vi "ADAM_Server_Channels.vi"() -> (0 "DAQ Error":errorcluster)   [LabVIEW 2015]
uses:
  ADAM Client/Sub VIs/ADAM Controls/Search_mode.ctl
  <vilib>/Analysis/baseanly.llb/Mean (DBL).vi
  Globals/Meas_global.vi
  Globals/Trav_pos_global.vi
  <vilib>/Analysis/NI_AALBase.lvlib
panel:
  out "Waveform Graph":dbl[][](graph)
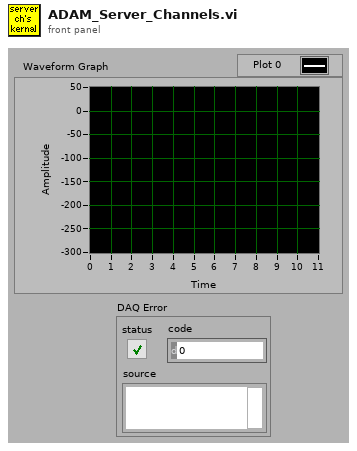
[diagram p1: front panel]
types:
  T1 = typedef "Analysis_info_cluster.ctl" = cluster{"Colour":u32, "Inst type":T2, "Inst name":string, "Symbol":string, "Code name":string, "Extra Info":string, "Inst Array":T3, "Extra Titles":string[], "Extra Values":string[], "U":dbl, "u^2":dbl, "u^3":dbl, "u^4":dbl, "Skew_u":dbl, "Kurt_u":dbl, "Sd Error in Mean":dbl, "% u'/U":dbl, "X":dbl, "Y":dbl, "Z":dbl, "Timescale integral to 25%":dbl, "Sd Error in Variance":dbl, "Calib File":path, "Calib Constants":dbl[], "Output Position":bool, "Full Stats":bool, "Av Sampling Rate":dbl, "Av No of Samples":dbl, "Total Meas Time (s)":dbl, "ADAM Ch Name":string}
  T2 = typedef "Inst_type.ctl" = enum16{"Propeller anemometer", "Raw voltage", "Pressure Transducer", "Pitot-static tube", "Preston tube", "Hot wire", "Cross wire 1", "Cross wire 2", "Generic Linear", "Generic Polynomial", "Generic BackPoly", "Fast FID", "Thermocouple", "Cold wire", "Pulsed Wire", "LDA Vel", "LDA Tran time", "LDA Arr time", "Microphone"}
  T3 = typedef "Instrument_Array.ctl" = enum16{"PWA", "LDA", "Analogue"}
  T4 = typedef "Search_mode.ctl" = enum16{"Between times", "All Times"}
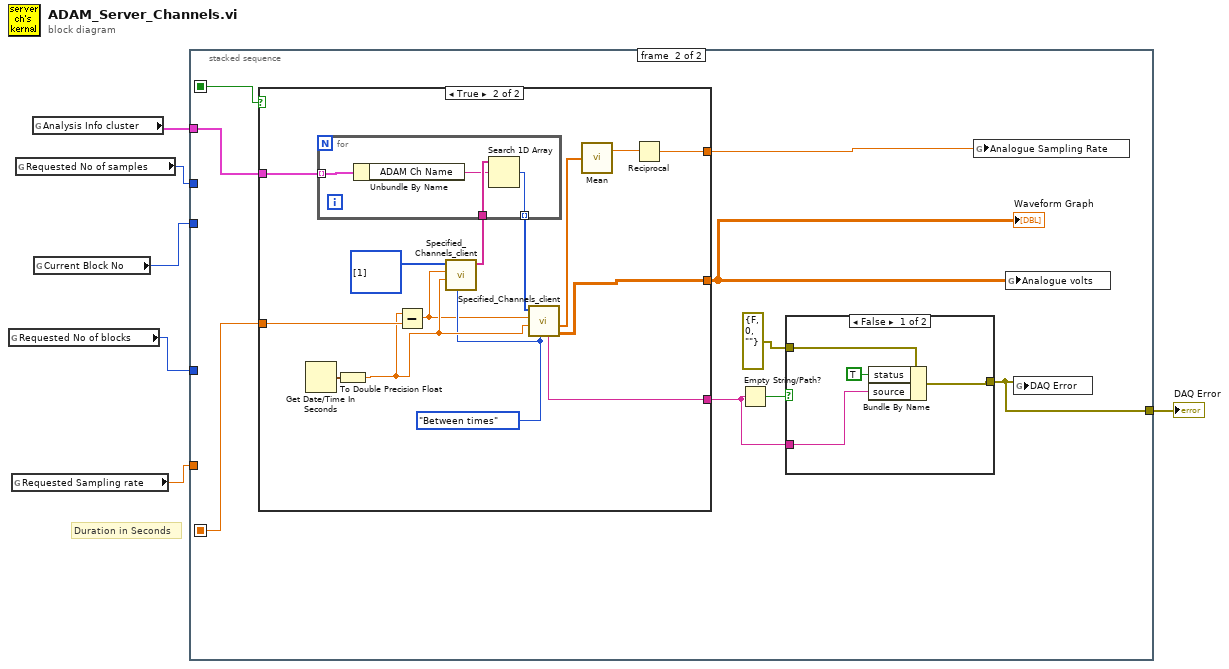
[diagram p0: block diagram]
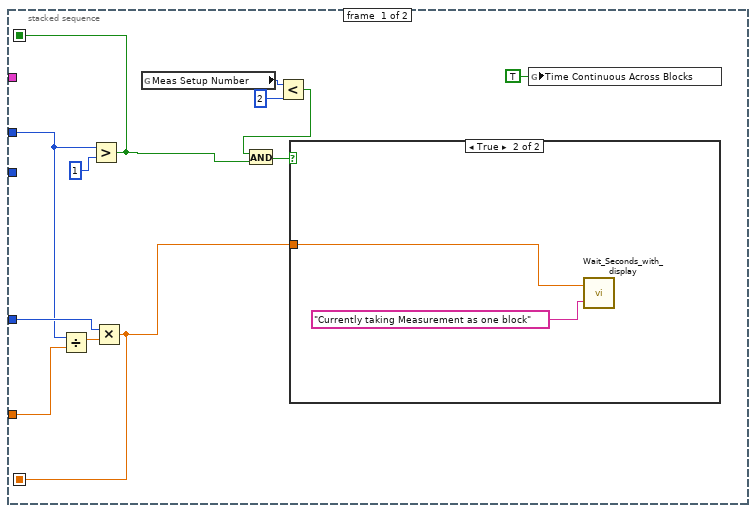
[diagram p2: hidden frame]
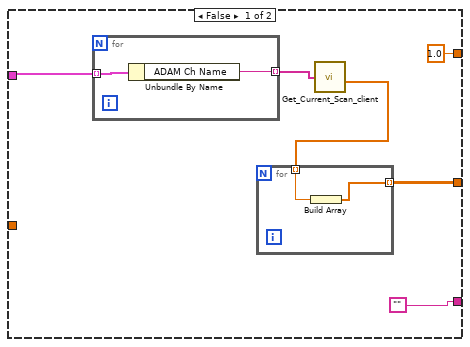
[diagram p4: hidden frame]
diagram:
  # "Duration in Seconds"
  n1 = global read "Meas_global.vi" "Requested No of blocks"() -> (w2:i32)
  n2 = global read "Meas_global.vi" "Requested Sampling rate"() -> (w5:dbl)
  n3 = global read "Meas_global.vi" "Requested No of samples"() -> (w6:i32)
  n4 = global read "Meas_global.vi" "Analysis Info cluster"() -> (w3:T1[])
  n5 = global read "Meas_global.vi" "Current Block No"() -> (w4:i32)
  n6 = stacked-sequence {
    seq-local: [w15 _] -> [_ w29]
    seq-local: [w9 _] -> [_ w22]
    tunnel: w6 -> [w14 _]
    tunnel: w4 -> [_ _]
    tunnel: w3 -> [_ w27]
    tunnel: w5 -> [w18 _]
    tunnel: w2 -> [w16 _]
    tunnel: [_ w21] -> w1
    frame #0 {
      n7 = Divide(x=w14, y=w18) -> (x/y=w17:dbl)
      n8 = Greater?(x=w14, y=1) -> (0:w9:bool)
      n9 = Multiply(x=w16, y=w17) -> (x*y=w15:dbl)
      n10 = global read "Trav_pos_global.vi" "Meas Setup Number"() -> (w12:i32)
      n11 = Less?(x=w12, y=2) -> (x < y?=w10:bool)
      n12 = And(x=w10, y=w9) -> (x .and. y?=w8:bool)
      n13 = case shown="True" w8 {
        tunnel: w15 -> [_ w19]
        frame False {
        }
        frame True {
          n14 = call "Wait_Seconds_with_display.vi"("Message"="Currently taking Measurement as one block", "Seconds to wait"=w19) -> ()  [unwired: 2 out]
        }
      }
      n15 = global write "Meas_global.vi" "Time Continuous Across Blocks"(TRUE ("Time Continuous across Blocks")) -> ()
    }
    frame #1 {
      n16 = case shown="True" w22 {
        tunnel: w29 -> [_ w52]
        tunnel: [w32 w45] -> w28
        tunnel: w27 -> [w35 w44]
        tunnel: [1.0 w41] -> w26
        tunnel: ["" w40] -> w23
        frame False {
          n17 = for {
            tunnel: w35 -> [w39] mode=indexing
            tunnel: [w38] -> w34 mode=indexing
            n18 = Unbundle By Name(w39) -> ("ADAM Ch Name"=w38:string)
          }
          n19 = call "Get_Current_Scan_client.vi"("ADAM Ch Names"=w34) -> ("Numerical Values"=w33:dbl[])  [unwired: 1 in, 2 out]
          n20 = for {
            tunnel: w33 -> [w37] mode=indexing
            tunnel: [w36] -> w32 mode=indexing
            n21 = Build Array(w37) -> (w36:dbl[])
          }
        }
        frame True {
          w47 = Search_mode."Between times" ("Mode")
          n22 = Get Date/Time In Seconds() -> (seconds since 1Jan1904=w53:timestamp)
          n23 = To Double Precision Float(number=w53) -> (double precision float=w51:dbl)
          n24 = Subtract(x=w51, y=w52) -> (x-y=w46:dbl)
          n25 = call "Specified_Channels_client.vi"("Mode"=w47, "End time"=w51, "Start time"=w46, "ADAM Index array"=i32[] [1]) -> ("All Active Ch Names"=w49:string[])  [unwired: 1 in, 6 out]
          n26 = for {
            tunnel: w44 -> [w57] mode=indexing
            tunnel: w49 -> [w56]
            tunnel: [w54] -> w48 mode=indexing
            n27 = Unbundle By Name(w57) -> ("ADAM Ch Name"=w55:string)
            n28 = Search 1D Array(1D array=w56, element=w55) -> (index of element=w54:i32)  [unwired: 1 out]
          }
          n29 = call "Specified_Channels_client.vi"("Mode"=w47, "End time"=w51, "Start time"=w46, "ADAM Index array"=w48) -> ("Output array"=w45:dbl[][], "Averaging Period"=w43:dbl[], "Messages"=w40:string)  [unwired: 1 in, 4 out]
          n30 = call-poly <vilib>:"Mean.vi"("X"=w43) -> ("mean"=w42:dbl)  [unwired: 1 out]
          n31 = Reciprocal(x=w42) -> (1/x=w41:dbl)
        }
      }
      "Waveform Graph" <- w28
      n32 = Empty String/Path?(string/path=w23) -> (empty?=w25:bool)
      n33 = case shown="False" w25 {
        tunnel: errorcluster {"status"=FALSE, "code"=0, "source"=""} ("DAQ Error") -> [w61 w62]
        tunnel: [w60 w62] -> w21
        tunnel: w23 -> [w58 _]
        frame False {
          n34 = Bundle By Name(cluster=w61, "status"=TRUE, "source"=w58) -> (w60:errorcluster)
        }
        frame True {
        }
      }
      n35 = global write "Meas_global.vi" "Analogue Sampling Rate"(w26) -> ()
      n36 = global write "Meas_global.vi" "Analogue volts"(w28) -> ()
      n37 = global write "Meas_global.vi" "DAQ Error"(w21) -> ()
    }
  }
  "DAQ Error" <- w1
